vi "Cluster Get Datatype From Variant.vi"(8 "Error In":errorcluster, 11 "cluster variant in":variant) -> (0 "Error Out":errorcluster, 3 "cluster elements datatypes":string[](array[string]))   [LabVIEW 2018]
uses:
  <vilib>/Utility/VariantDataType/VariantType.lvlib
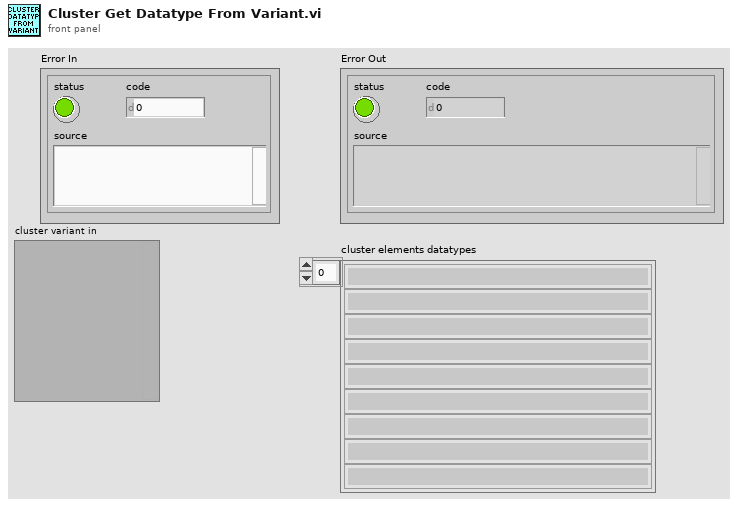
[diagram p1: front panel]
types:
  T1 = typedef "VariantType.lvlib/TypedefInfo.ctl" = cluster{"Name":string, "Timestamp":u32}
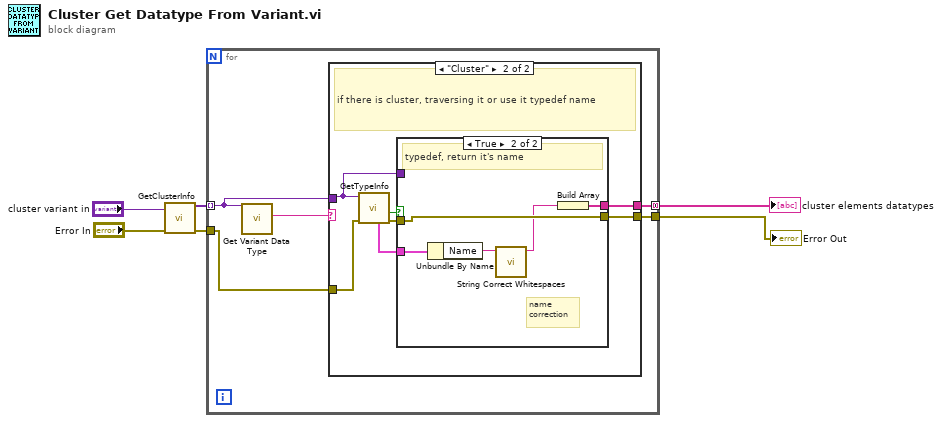
[diagram p0: block diagram]
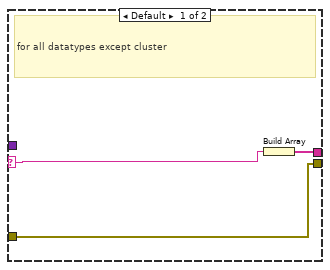
[diagram p2: hidden frame]
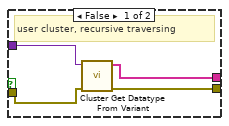
[diagram p3: hidden frame]
diagram:
  n1 = call <vilib>:"GetClusterInfo.vi"("error in (no error)"="Error In", "Variant"="cluster variant in") -> ("error out"=w2:errorcluster, "Cluster Elements"=w5:variant[])  [unwired: 8 in]
  n2 = for {
    tunnel: w5 -> [w11] mode=indexing
    tunnel: [w10] -> w4 mode=concatenating
    tunnel: w2 -> [w9]
    tunnel: [w8] -> w1
    n3 = call "Get Variant Data Type.vi"("Variant in"=w11) -> ("first data type"=w7:string)  [unwired: 9 in, 1 out]
    n4 = case shown="\"Cluster\"" w7 {
      selector: w7 -> [w12 _]
      tunnel: w11 -> [_ w18]
      tunnel: [w14 w19] -> w10
      tunnel: w9 -> [w13 w17]
      tunnel: [w13 w15] -> w8
      frame Default {
        # "for all datatypes except cluster"
        n5 = Build Array(w12) -> (w14:string[])
      }
      frame "Cluster" {
        # "if there is cluster, traversing it or use it typedef name"
        n6 = call <vilib>:"GetTypeInfo.vi"("error in (no error)"=w17, "Variant"=w18) -> ("error out"=w16:errorcluster, "HasTypedef"=w21:bool, "TypedefInfo"=w20:T1)  [unwired: 5 in, 2 out]
        n7 = case shown="True" w21 {
          tunnel: w20 -> [_ w30]
          tunnel: [w24 w29] -> w19
          tunnel: w18 -> [w25 _]
          tunnel: w16 -> [w23 w28]
          tunnel: [w22 w28] -> w15
          frame False {
            # "user cluster, recursive traversing"
            n8 = call "Cluster Get Datatype From Variant.vi"("Error In"=w23, "cluster variant in"=w25) -> ("Error Out"=w22:errorcluster, "cluster elements datatypes"=w24:string[])  [unwired: 8 in]
          }
          frame True {
            # "name correction"
            # "typedef, return it's name"
            n9 = Unbundle By Name(w30) -> ("Name"=w27:string)
            n10 = call "String Correct Whitespaces.vi"("String in"=w27) -> ("String out"=w26:string)  [unwired: 10 in]
            n11 = Build Array(w26) -> (w29:string[])
          }
        }
      }
    }
  }
  "Error Out" <- w1
  "cluster elements datatypes" <- w4
